vi "GreeterService GetFeature.vi"(3 "error in (no error)":errorcluster, 4 "gRPCid in":T1, 5 "DNL_LabVIEW Object in":refnum<class "GreeterServiceImpl.lvclass">) -> (0 "error out":errorcluster, 1 "gRPCid out":T1, 2 "DNL_LabVIEW Object out":refnum<class "GreeterServiceImpl.lvclass">)   [LabVIEW 2019, in "UserCode_server.lvlib" / "GreeterServiceImpl.lvclass"]
uses:
  GreeterServiceImpl.lvclass
  <vilib>/gRPC/LabVIEW gRPC Library/Shared/grpcId.ctl
  Generated_server/RPC Messages/Greeter_res.ctl
  Generated_server/RPC Messages/Greeter_res_res_oneof/Greeter_res_res_oneof.lvclass
  Generated_server/RPC Messages/Greeter_req_req_oneof/Greeter_req_req_oneof.lvclass/Greeter_req_req_oneof.ctl
  Generated_server/RPC Messages/Greeter_res_res_oneof/Greeter_res_res_oneof.lvclass/Greeter_res_res_oneof.ctl
  Generated_server/RPC Service/GreeterService/GreeterService.lvclass
  Generated_server/RPC Messages/Greeter_req_req_oneof/Greeter_req_req_oneof.lvclass
  Generated_server/Generated_server.lvlib
  <vilib>/gRPC/LabVIEW gRPC Library/grpc-lvsupport-release.lvlib
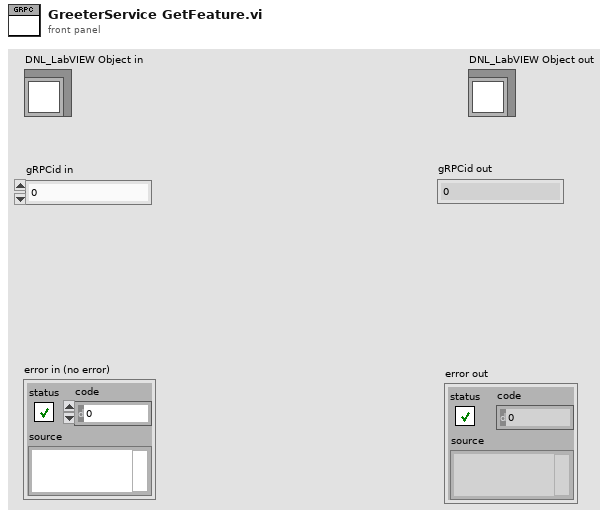
[diagram p1: front panel]
types:
  T1 = typedef "grpc-lvsupport-release.lvlib/grpcId.ctl" = u64
  T2 = typedef "Generated_server.lvlib/Greeter_res.ctl" = cluster{"res_id":i32, "Greeter_res_res_oneof":refnum<class "Greeter_res_res_oneof.lvclass">}
  T3 = typedef "Generated_server.lvlib/Greeter_req.ctl" = cluster{"req_id":i32, "Greeter_req_req_oneof":refnum<class "Greeter_req_req_oneof.lvclass">}
  T4 = typedef "Generated_server.lvlib/Greeter_MessageA.ctl" = cluster{"data_a1":string}
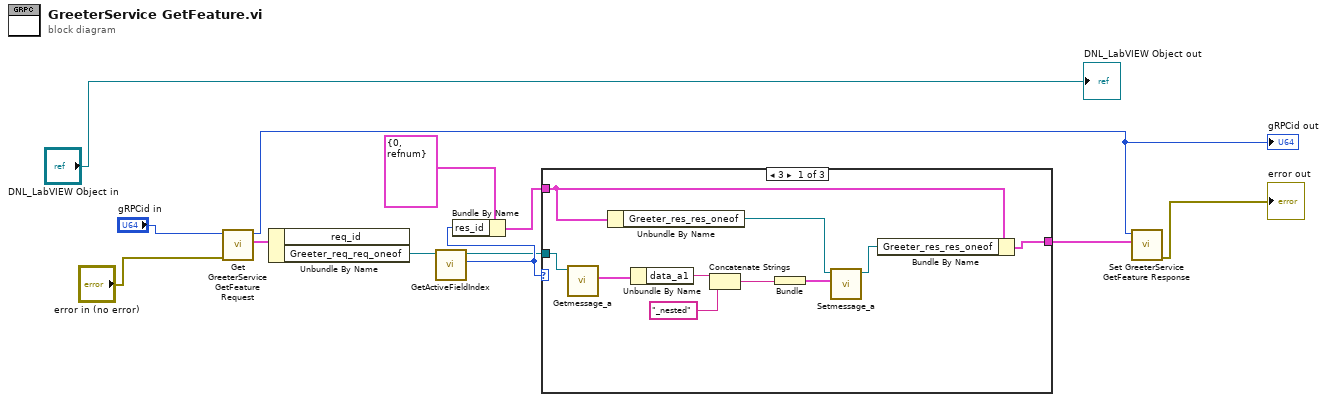
[diagram p0: block diagram]
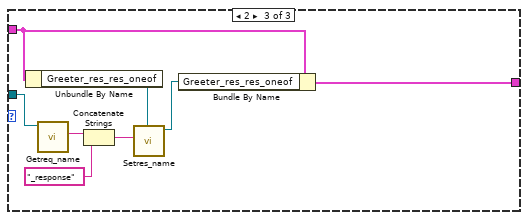
[diagram p3: hidden frame]
diagram:
  n1 = call "Get GreeterService GetFeature Request.vi"("error in (no error)"="error in (no error)", "gRPCid"="gRPCid in") -> ("Message Data"=w12:T3, "gRPCid out"=w2:T1)  [unwired: 7 in, 1 out]
  "gRPCid out" <- w2
  n2 = Unbundle By Name(w12) -> ("Greeter_req_req_oneof"=w11:refnum<class "Greeter_req_req_oneof.lvclass">)  [unwired: 1 out]
  n3 = call "GetActiveFieldIndex.vi"("OneOfTemplate in"=w11) -> ("Active Field Index"=w10:i32, "OneOfTemplate out"=w8:refnum<class "Greeter_req_req_oneof.lvclass">)  [unwired: 8 in, 1 out]
  n4 = Bundle By Name(cluster=T2 {"res_id"=0, "Greeter_res_res_oneof"=refnum} ("Greeter_res"), "res_id"=w10) -> (w9:T2)
  n5 = case shown="3" w10 {
    tunnel: w9 -> [w15 w23 w27]
    tunnel: w8 -> [w22 _ w31]
    tunnel: [w13 w23 w24] -> w6
    frame 3 {
      n6 = call "Getmessage_a.vi"("OneOfTemplate in"=w22) -> ("Get_Val"=w21:T4)  [unwired: 8 in, 2 out]
      n7 = Unbundle By Name(w15) -> ("Greeter_res_res_oneof"=w16:refnum<class "Greeter_res_res_oneof.lvclass">)
      n8 = Unbundle By Name(w21) -> ("data_a1"=w20:string)
      n9 = Concatenate Strings(w20, "_nested" ("string")) -> (w18:string)
      n10 = Bundle(w18) -> (w17:cluster{string})  [unwired: 1 in]
      n11 = call "Setmessage_a.vi"("Set_Val"=w17, "OneOfTemplate in"=w16) -> ("OneOfTemplate out"=w14:refnum<class "Greeter_res_res_oneof.lvclass">)  [unwired: 8 in, 1 out]
      n12 = Bundle By Name(cluster=w15, "Greeter_res_res_oneof"=w14) -> (w13:T2)
    }
    frame 0, Default {
    }
    frame 2 {
      n13 = Unbundle By Name(w27) -> ("Greeter_res_res_oneof"=w26:refnum<class "Greeter_res_res_oneof.lvclass">)
      n14 = call "Getreq_name.vi"("OneOfTemplate in"=w31) -> ("Get_Val"=w30:string)  [unwired: 8 in, 2 out]
      n15 = Concatenate Strings(w30, "_response" ("string")) -> (w28:string)
      n16 = call "Setres_name.vi"("Set_Val"=w28, "OneOfTemplate in"=w26) -> ("OneOfTemplate out"=w25:refnum<class "Greeter_res_res_oneof.lvclass">)  [unwired: 8 in, 1 out]
      n17 = Bundle By Name(cluster=w27, "Greeter_res_res_oneof"=w25) -> (w24:T2)
    }
  }
  n18 = call "Set GreeterService GetFeature Response.vi"("Message Data"=w6, "gRPCid in"=w2) -> ("error out"=→"error out":errorcluster)  [unwired: 9 in]
  "DNL_LabVIEW Object out" <- "DNL_LabVIEW Object in"
